vi "Read.vi"(8 "error in (no error)":errorcluster, 11 "Save Var Command Config in":refnum<class "Save Var Command Config.lvclass">) -> (0 "error out":errorcluster, 1 "Channel Name":string, 2 "Var Name":string, 3 "Save Var Command Config out":refnum<class "Save Var Command Config.lvclass">)   [LabVIEW 2020, in "VolatusSeqConfig.lvlib" / "Save Var Command Config.lvclass"]
uses:
  Save Var Command Config.lvclass
  Save Var Command Config.lvclass/Save Var Command Config.ctl
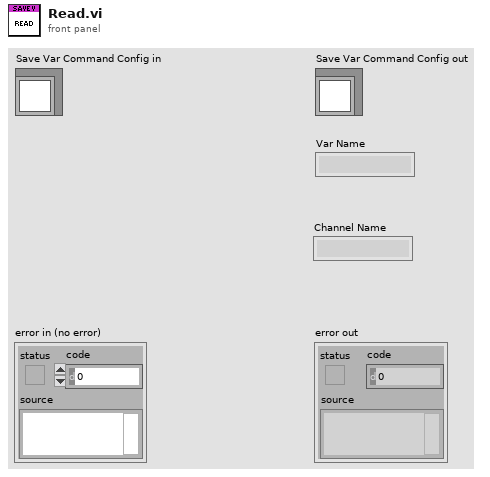
[diagram p1: front panel]
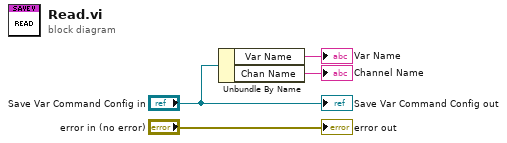
[diagram p0: block diagram]
diagram:
  n1 = Unbundle By Name("Save Var Command Config in") -> ("Var Name"=→"Var Name":string, "Chan Name"=→"Channel Name":string)
  "error out" <- "error in (no error)"
  "Save Var Command Config out" <- "Save Var Command Config in"
